vi "isFacadeConnected.vi"(8 "error in (no error)":errorcluster, 11 "SMOFacade in":refnum<class "SMOFacade.lvclass">) -> (0 "error out":errorcluster, 2 "isConnected":bool, 3 "SMOFacade out":refnum<class "SMOFacade.lvclass">)   [LabVIEW 2021, in "smo.lvlib" / "SMOFacade.lvclass"]
uses:
  SMOFacade.lvclass
  SMOFacade.lvclass/SMOFacade.ctl
  SMO/SMO.lvclass
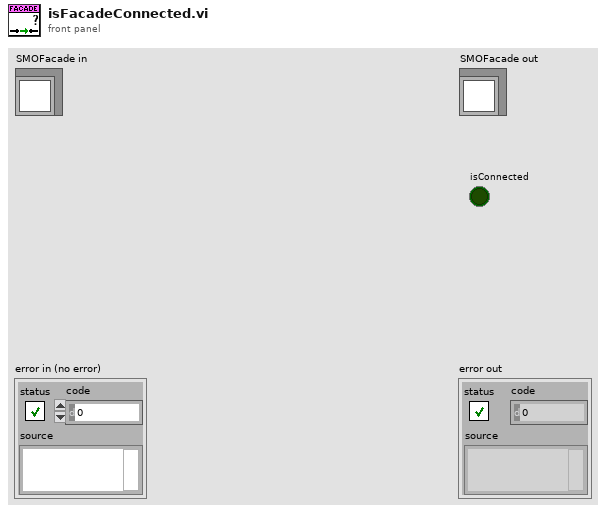
[diagram p1: front panel]
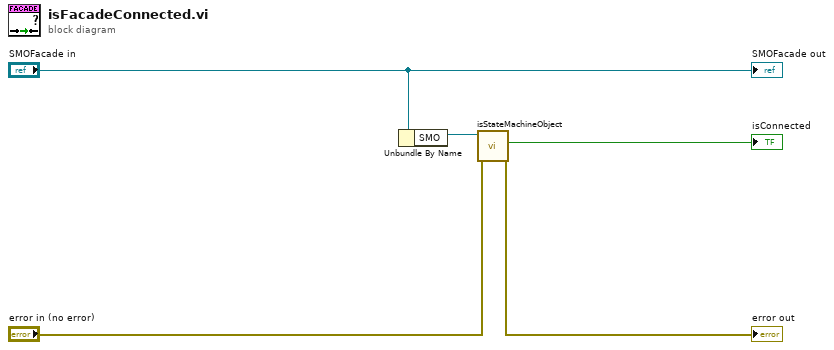
[diagram p0: block diagram]
diagram:
  n1 = Unbundle By Name("SMOFacade in") -> ("SMO"=w4:refnum<class "SMO.lvclass">)
  n2 = call "isStateMachineObject.vi"("error in (no error)"="error in (no error)", "SMO"=w4) -> ("error out"=→"error out":errorcluster, "is SMO?"=→"isConnected":bool)  [unwired: 7 in, 1 out]
  "SMOFacade out" <- "SMOFacade in"
